vi "Chart_Data_Packer.vi"(0 "DataCluster":T1={"Core"={"Current VI Reference"=refnum, "Close Panel on Exit?"=FALSE, "Exit"=FALSE, "Initialized?"=FALSE}, "Connections"={"cDAQ Therm"={"Task"="", "Connected"=FALSE, "Active"=FALSE}, "cDAQ Voltage"={"Task"="", "Connected"=FALSE, "Active"=FALSE}, "cDAQ ID"="", "Camera"={"Session"="", "Connected"=FALSE, "Active"=FALSE, "Placeholder"=refnum}, "PSU"={"Port"="", "Connected"=FALSE, "Active"=FALSE}}, "Data Acquisition"={"Setup"={"Label"="", "Operator"="", "Notes"="", "TempGrad"=1.0, "TargetTemp"=1.0, "Sample Volume"=1.0}, "Camera"={"Image"=refnum, "Save Image"=refnum, "Image Frequency"=20, "Rectangle"={"Left"=0, "Top"=0, "Right"=0, "Bottom"=0, "Rotation"=0.0}, "Calibration"={"Top Left"={"X"=0.0, "Y"=0.0}, "Top Right"={"X"=0.0, "Y"=0.0}, "Bottom Left"={"X"=0.0, "Y"=0.0}, "Bottom Right"={"X"=0.0, "Y"=0.0}, "Fixpoint"={"X"=0.0, "Y"=0.0}, "Scan Area"=0.0, "Fixpoint Area"=0.0, "Well Pixels"=[], "Valid"=FALSE}, "FocusPos"=0, "Display Mapping"=10}, "Thermistor"={"Sample Size"=1, "Calibration"={"B0.100"=[], "R25"=[], "c"=[], "State"=[], "V_S"=5.0, "R_S"=100.0}, "Timing Mode"=14713}, "Partition"={"Data"=[], "Cell Label"="", "Cell Color"=0, "Height"=10, "Width"=16, "Grid"=[]}, "Queue"={"Size"=1, "Queue"=refnum}, "Sample Rate"=1, "Active"=FALSE, "Ready"=FALSE, "Graph Mode"=0}, "Control"={"Sample Rate"=1, "PID gains"={"proportional gain (Kc)"=1.0, "integral time (Ti, min)"=0.01, "derivative time (Td, min)"=0.0}}} {"Control"."PID gains"."derivative time (Td, min)" format="%.3f"; "Control"."PID gains"."integral time (Ti, min)" format="%.3f"; "Control"."PID gains"."proportional gain (Kc)" format="%.3f"; "Control"."Sample Rate" min=1 max=20 step=1 format="%.0f Samples/sec"; "Data Acquisition"."Graph Mode" items=["Thermistor Temperature", "Camera Temperature"]; "Data Acquisition"."Thermistor"."Timing Mode" items=["Automatic"=16097, "High Resolution"=10195, "High Speed"=14712, "Best 50 Hz Rejection"=14713, "Best 60 Hz Rejection"=14714, "Custom"=10137]; "Data Acquisition"."Thermistor"."Calibration"."R_S" min=0.1 max=1000.0 format="%#_g kOhm"; "Data Acquisition"."Thermistor"."Calibration"."V_S" min=5.0 max=48.0 format="%#_g V"; "Data Acquisition"."Thermistor"."Calibration"."R25" min=0.1 max=1000.0 format="%#_g kOhm"; "Data Acquisition"."Thermistor"."Calibration"."B0.100" min=100.0 max=10000.0 format="%#_g K"; "Data Acquisition"."Thermistor"."Sample Size" min=1 max=200; "Data Acquisition"."Sample Rate" min=20 max=240 format="%.0f samples/min"; "Data Acquisition"."Queue"."Size" min=1 max=200; "Data Acquisition"."Camera"."Display Mapping" items=["Default"=10, "Most Significant Bits"=11, "Full Dynamic"=12, "Downshift"=13, "Given Range"=14, "90% Dynamic"=15, "Given Percent Range"=16]; "Data Acquisition"."Camera"."Calibration"."Fixpoint"."Y" format="%.2f"; "Data Acquisition"."Camera"."Calibration"."Fixpoint"."X" format="%.2f"; "Data Acquisition"."Camera"."Calibration"."Top Left"."Y" format="%.2f"; "Data Acquisition"."Camera"."Calibration"."Top Left"."X" format="%.2f"; "Data Acquisition"."Camera"."Calibration"."Top Right"."Y" format="%.2f"; "Data Acquisition"."Camera"."Calibration"."Top Right"."X" format="%.2f"; "Data Acquisition"."Camera"."Calibration"."Bottom Left"."Y" format="%.2f"; "Data Acquisition"."Camera"."Calibration"."Bottom Left"."X" format="%.2f"; "Data Acquisition"."Camera"."Calibration"."Bottom Right"."Y" format="%.2f"; "Data Acquisition"."Camera"."Calibration"."Bottom Right"."X" format="%.2f"; "Data Acquisition"."Camera"."Rectangle"."Rotation" min=-90.0 max=90.0 step=1.0 format="%.2f"; "Data Acquisition"."Camera"."Rectangle"."Left" scale=0.0..1024.0; "Data Acquisition"."Camera"."Rectangle"."Right" scale=0.0..1024.0; "Data Acquisition"."Camera"."Image Frequency" min=1 max=60 step=1; "Data Acquisition"."Setup"."Sample Volume" min=0.0 max=500.0 format="%#_g µL"; "Data Acquisition"."Setup"."TargetTemp" min=-40.0 max=40.0 step=0.5 format="%#_g °C"; "Data Acquisition"."Setup"."TempGrad" min=-100.0 max=100.0 step=0.1 format="%#_g °C/min"}, 5 "Mean Temperature":dbl format="%0.2f", 7 "Temperatures":dbl[](array[numeric]), 9 "Temp Gradient":dbl, 11 "Data Cluster in":cluster{dbl[], dbl[], dbl[], dbl[], dbl[][]}, 12 "DAQ/Control":u16(ring)=1 items=["DAQ", "Control"]) -> (4 "Chart Data":waveform(dbl)[](array[waveform]), 6 "Gradients":waveform(dbl)[](array[waveform]), 8 "Temps":waveform(dbl)[](array[waveform]), 15 "Data Cluster":cluster{dbl[], dbl[], dbl[], dbl[], dbl[][]})   [LabVIEW 2020]
uses:
  DataCluster.ctl
  <vilib>/userdefined/High Color/IMAQdx.ctl
  <vilib>/vision/Image Controls.llb/IMAQ Image.ctl
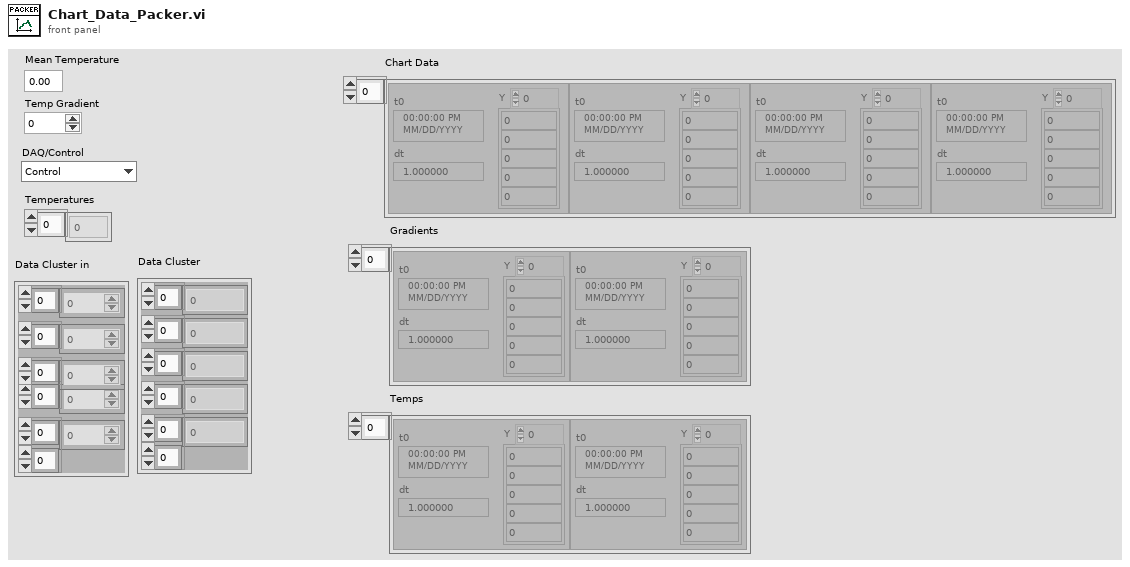
[diagram p1: front panel]
types:
  T1 = typedef "DataCluster.ctl" = cluster{"Core":cluster{"Current VI Reference":refnum<vi>, "Close Panel on Exit?":bool, "Exit":bool, "Initialized?":bool}, "Connections":cluster{"cDAQ Therm":cluster{"Task":refnum<k21>, "Connected":bool, "Active":bool}, "cDAQ Voltage":cluster{"Task":refnum<k21>, "Connected":bool, "Active":bool}, "cDAQ ID":string, "Camera":cluster{"Session":T2, "Connected":bool, "Active":bool, "Placeholder":T3}, "PSU":cluster{"Port":refnum<visa-resource-name>, "Connected":bool, "Active":bool}}, "Data Acquisition":cluster{"Setup":cluster{"Label":string, "Operator":string, "Notes":string, "TempGrad":dbl, "TargetTemp":dbl, "Sample Volume":dbl}, "Camera":cluster{"Image":T3, "Save Image":T3, "Image Frequency":i32, "Rectangle":T4, "Calibration":cluster{"Top Left":T5, "Top Right":T5, "Bottom Left":T5, "Bottom Right":T5, "Fixpoint":T5, "Scan Area":dbl, "Fixpoint Area":dbl, "Well Pixels":cluster{"X":i32, "Y":i32}[][], "Valid":bool}, "FocusPos":u32, "Display Mapping":u32}, "Thermistor":cluster{"Sample Size":i32, "Calibration":cluster{"B0.100":dbl[], "R25":dbl[], "c":dbl[][], "State":bool[], "V_S":dbl, "R_S":dbl}, "Timing Mode":i32}, "Partition":cluster{"Data":string[][], "Cell Label":string, "Cell Color":u32, "Height":i32, "Width":i32, "Grid":string[][]}, "Queue":cluster{"Size":i32, "Queue":refnum<queue>}, "Sample Rate":i32, "Active":bool, "Ready":bool, "Graph Mode":u16}, "Control":cluster{"Sample Rate":i32, "PID gains":cluster{"proportional gain (Kc)":dbl, "integral time (Ti, min)":dbl, "derivative time (Td, min)":dbl}}}
  T2 = typedef "IMAQdx.ctl" = refnum<k21>
  T3 = typedef "IMAQ Image.ctl" = refnum<image>
  T4 = typedef "IMAQ Rectangle" = cluster{"Left":i32, "Top":i32, "Right":i32, "Bottom":i32, "Rotation":dbl}
  T5 = typedef "IMAQ Point" = cluster{"X":sgl, "Y":sgl}
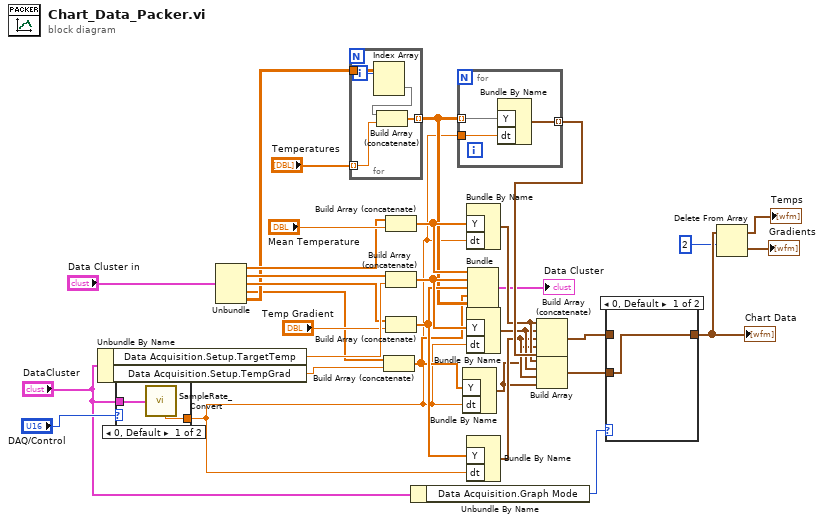
[diagram p0: block diagram]
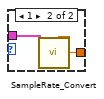
[diagram p3: hidden frame]
diagram:
  n1 = Unbundle By Name("DataCluster") -> ("Data Acquisition.Setup.TargetTemp"=w31:dbl, "Data Acquisition.Setup.TempGrad"=w12:dbl)
  n2 = case shown="0, Default" "DAQ/Control" {
    tunnel: [w33 w36] -> w6
    tunnel: "DataCluster" -> [w34 w35]
    frame 0, Default {
      n3 = call "SampleRate_Convert.vi"("DataCluster"=w34) -> ("Sample dt (s)"=w33:dbl)  [unwired: 5 in, 3 out]
    }
    frame 1 {
      n4 = call "SampleRate_Convert.vi"("DataCluster"=w35) -> ("Control Sample dt (s)"=w36:dbl)  [unwired: 5 in, 3 out]
    }
  }
  n5 = Unbundle("Data Cluster in") -> (w24:dbl[], w25:dbl[], w26:dbl[], w8:dbl[], w9:dbl[][])
  n6 = for {
    tunnel: "Temperatures" -> [w41] mode=indexing
    tunnel: [w40] -> w21 mode=indexing
    tunnel: w9 -> [w38]
    i -> [w39]
    n7 = Index Array(array=w38, index (row)=w39) -> (element=w37:dbl[])  [unwired: 1 in]
    n8 = Build Array (concatenate)(w37, w41) -> (w40:dbl[])
  }
  n9 = Build Array (concatenate)(w8, w12) -> (w7:dbl[])
  n10 = Build Array (concatenate)(w24, "Mean Temperature") -> (w29:dbl[])
  n11 = Build Array (concatenate)(w25, w31) -> (w30:dbl[])
  n12 = Build Array (concatenate)(w26, "Temp Gradient") -> (w27:dbl[])
  n13 = Unbundle By Name("DataCluster") -> ("Data Acquisition.Graph Mode"=w18:u16)
  n14 = for {
    tunnel: w21 -> [w44] mode=indexing
    tunnel: w6 -> [w43]
    tunnel: [w42] -> w20 mode=indexing
    n15 = Bundle By Name("Y"=w44, "dt"=w43) -> (w42:waveform(dbl))  [unwired: 1 in]
  }
  n16 = Bundle By Name("Y"=w7, "dt"=w6) -> (w5:waveform(dbl))  [unwired: 1 in]
  n17 = Bundle By Name("Y"=w29, "dt"=w6) -> (w17:waveform(dbl))  [unwired: 1 in]
  n18 = Bundle By Name("Y"=w30, "dt"=w6) -> (w16:waveform(dbl))  [unwired: 1 in]
  n19 = Bundle By Name("Y"=w27, "dt"=w6) -> (w15:waveform(dbl))  [unwired: 1 in]
  n20 = Bundle(w29, w30, w27, w7, w21) -> (→"Data Cluster":cluster{dbl[], dbl[], dbl[], dbl[], dbl[][]})  [unwired: 1 in]
  n21 = Build Array (concatenate)(w17, w16, w15, w5, w20) -> (w14:waveform(dbl)[])
  n22 = Build Array(w17, w16, w15, w5) -> (w13:waveform(dbl)[])
  n23 = case shown="0, Default" w18 {
    tunnel: w14 -> [_ w46]
    tunnel: w13 -> [w45 _]
    tunnel: [w45 w46] -> w4
    frame 0, Default {
    }
    frame 1 {
    }
  }
  "Chart Data" <- w4
  n24 = Delete From Array(array=w4, length=2) -> (deleted portion=→"Gradients":waveform(dbl)[], array with subset deleted=→"Temps":waveform(dbl)[])  [unwired: 1 in]
